vi "move.vi"(8 "error in (no error)":errorcluster, 11 "DL090602SutterMP285Stage in":refnum<class "StageDL090602SutterMP285.lvclass">) -> (0 "error out":errorcluster, 3 "DL090602SutterMP285Stage out":refnum<class "StageDL090602SutterMP285.lvclass">)   [LabVIEW 2010, in "StageDL090602SutterMP285.lvclass"]
uses:
  StageDL090602SutterMP285.lvclass
  StageDL090409Scaffold/StageDL090409Scaffold/StageDL090409Scaffold.lvclass
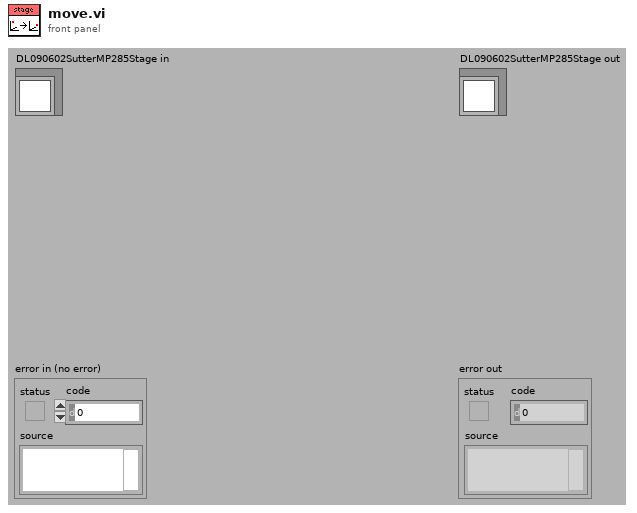
[diagram p1: front panel]
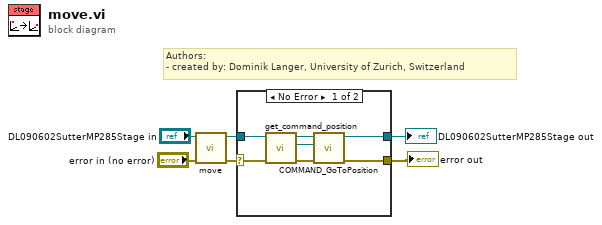
[diagram p0: block diagram]
diagram:
  # "Authors: \n- created by: Dominik Langer, University of Zurich, Switzerland"
  n1 = call-parent "move.vi"("error in (no error)"="error in (no error)", "DL090409StageScaffold in"="DL090602SutterMP285Stage in") -> ("error out"=w3:errorcluster, "DL090409StageScaffold out"=w1:refnum<class "StageDL090602SutterMP285.lvclass">)  [unwired: 8 out]
  n2 = case shown="No Error" w3 {
    selector: w3 -> [w13 w15]
    tunnel: [w8 w15] -> w6
    tunnel: [w7 w14] -> w5
    tunnel: w1 -> [w12 w14]
    frame No Error {
      n3 = call-dynamic "get_command_position.vi"("error in (no error)"=w13, "DL090409StageScaffold.lvclass in"=w12) -> ("error out"=w11:errorcluster, "SpaceVector.lvclass"=w10:refnum<class "SpaceVector.lvclass">, "DL090409StageScaffold.lvclass out"=w9:refnum<class "StageDL090602SutterMP285.lvclass">)  [unwired: 7 out]
      n4 = call-dynamic "COMMAND_GoToPosition.vi"("error in (no error)"=w11, "target  position"=w10, "StageDL090602SutterMP285 in"=w9) -> ("error out"=w8:errorcluster, "StageDL090602SutterMP285 out"=w7:refnum<class "StageDL090602SutterMP285.lvclass">)  [unwired: 7 in]
    }
    frame Error {
    }
  }
  "error out" <- w6
  "DL090602SutterMP285Stage out" <- w5
